vi "Get Wavelength or Frequency.vi"(8 "error in (no error)":errorcluster, 10 "return units (wavelength - air)":T1(ring)=enum."wavelength - air (nm)") -> (0 "error out":errorcluster, 2 "result":dbl)   [LabVIEW 2012, in "HighFinesse WS5.lvlib"]
doc: "Gets the current wavelenth (nm) or frequency (THz) from the wavelength meter. Maximum repetition rate appears to be 0.03 ms per reading (~30 kHz)."
uses:
  HighFinesse WS5.lvlib
  wlmData.dll
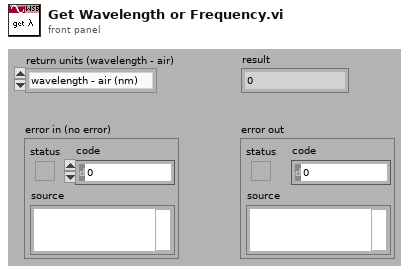
[diagram p1: front panel]
types:
  T1 = enum16{"wavelength - vac (nm)", "wavelength - air (nm)", "frequency (THz)", "wavenumber (1/cm)", "photon energy (eV)"}
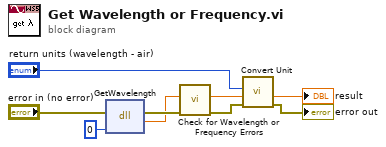
[diagram p0: block diagram]
diagram:
  n1 = dll-call lib="C:/LabView/Instruments/Wavelength meter/HighFinesse WS5/wlmData.dll" fn="GetWavelength"(error in="error in (no error)", "F"=0) -> (error out=w8:errorcluster, "return type"=w7:dbl)  [unwired: 3 in, 1 out]
  n2 = call "Check for Wavelength or Frequency Errors.vi"("error in (no error)"=w8, "return code"=w7) -> ("error out"=w5:errorcluster, "return code out"=w6:dbl)  [unwired: 8 out]
  n3 = call "Convert Unit.vi"("error in (no error)"=w5, "value"=w6, "unit to (air)"="return units (wavelength - air)") -> ("error out"=→"error out":errorcluster, "value out"=→"result":dbl)  [unwired: 1 in, 6 out]
